vi "Query Trace Data.vi"(8 "error in (no error)":errorcluster, 10 "Trace Number":u8=1, 11 "VNA-PNA in":refnum<class "VNA-PNA.lvclass">) -> (0 "error out":errorcluster, 1 "Data":dbl[](array[numeric]), 2 "Frequency":dbl[](array[numeric]), 3 "VNA-PNA out":refnum<class "VNA-PNA.lvclass">)   [LabVIEW 2020, in "VNA-PNA.lvclass"]
doc: "Query the active trace data.\nIt returns both x and y data"
uses:
  VNA-PNA.lvclass
  C:/Sandbox/RF Bench/Source Code/WiSpry Test Framework/Instruments/Instrument.lvclass
  C:/Sandbox/RF Bench/Source Code/WiSpry Test Framework/Instruments/Vector Network Analyzer/Vector Network Analyzer.lvclass
  Vector Network Analyzer.lvclass/Vector Network Analyzer.ctl
  Instrument.lvclass/Instrument.ctl
  Instrument.lvclass
  Vector Network Analyzer.lvclass
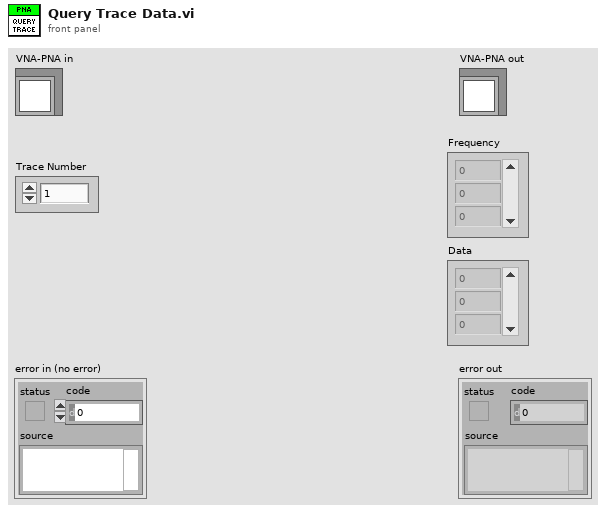
[diagram p1: front panel]
types:
  T1 = enum16{"big-endian, network order", "native, host order", "little-endian"}
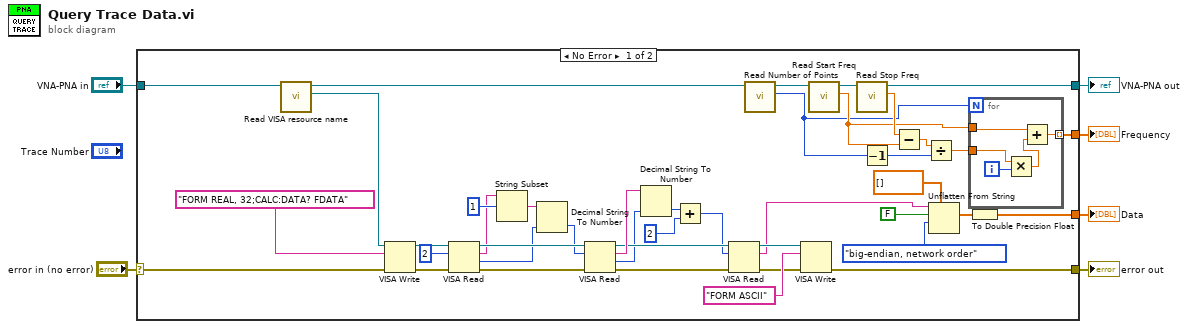
[diagram p0: block diagram]
diagram:
  n1 = case shown="No Error" "error in (no error)" {
    selector: "error in (no error)" -> [w48 w55]
    tunnel: [w29 w55] -> w3
    tunnel: [w36 w54] -> w4
    tunnel: [w31 _] -> w1
    tunnel: [w14 _] -> w2
    tunnel: "VNA-PNA in" -> [w7 w54]
    frame No Error {
      n2 = call "Read VISA resource name.vi"("Instrument in"=w7) -> ("VISA resource name"=w47:refnum<visa-resource-name>, "Instrument out"=w39:refnum<class "VNA-PNA.lvclass">)  [unwired: 9 in]
      n3 = VISA Write(VISA resource name=w47, write buffer="FORM REAL, 32;CALC:DATA? FDATA" ("initial string"), error in (no error)=w48) -> (VISA resource name out=w45:refnum<visa-resource-name>, error out=w46:errorcluster)  [unwired: 1 out]
      n4 = VISA Read(VISA resource name=w45, byte count=u32 2, error in (no error)=w46) -> (VISA resource name out=w42:refnum<visa-resource-name>, read buffer=w20:string, return count=w41:u32, error out=w43:errorcluster)
      n5 = String Subset(string=w20, offset (0)=1) -> (substring=w22:string)  [unwired: 1 in]
      n6 = Decimal String To Number(string=w22, default (0L)=w41) -> (number=w12:u32)  [unwired: 1 in, 1 out]
      n7 = VISA Read(VISA resource name=w42, byte count=w12, error in (no error)=w43) -> (VISA resource name out=w27:refnum<visa-resource-name>, read buffer=w28:string, return count=w19:u32, error out=w26:errorcluster)
      n8 = Decimal String To Number(string=w28, default (0L)=w19) -> (number=w23:u32)  [unwired: 1 in, 1 out]
      n9 = Add(x=w23, y=u32 2) -> (x+y=w11:u32)
      n10 = VISA Read(VISA resource name=w27, byte count=w11, error in (no error)=w26) -> (VISA resource name out=w24:refnum<visa-resource-name>, read buffer=w18:string, error out=w25:errorcluster)  [unwired: 1 out]
      n11 = call "Read Number of Points.vi"("Vector Network Analyzer in"=w39) -> ("Number of Points"=w8:i32, "Vector Network Analyzer out"=w38:refnum<class "VNA-PNA.lvclass">)  [unwired: 9 in]
      n12 = VISA Write(VISA resource name=w24, write buffer="FORM ASCII", error in (no error)=w25) -> (error out=w29:errorcluster)  [unwired: 2 out]
      n13 = call "Read Start Freq.vi"("Vector Network Analyzer in"=w38) -> ("Start Freq"=w33:dbl, "Vector Network Analyzer out"=w37:refnum<class "VNA-PNA.lvclass">)  [unwired: 9 in]
      n14 = call "Read Stop Freq.vi"("Vector Network Analyzer in"=w37) -> ("Stop Freq"=w35:dbl, "Vector Network Analyzer out"=w36:refnum<class "VNA-PNA.lvclass">)  [unwired: 9 in]
      n15 = Decrement(x=w8) -> (x-1=w9:i32)
      n16 = Subtract(x=w35, y=w33) -> (x-y=w34:dbl)
      n17 = Divide(x=w34, y=w9) -> (x/y=w32:dbl)
      n18 = Unflatten From String(type=sgl[] [], binary string=w18, data includes array or string size? (T)=FALSE, byte order (0:big-endian, network order)=T1."big-endian, network order") -> (value=w15:sgl[])  [unwired: 1 in, 2 out]
      n19 = for {
        N: w8 -> [_]
        tunnel: w33 -> [w50]
        tunnel: w32 -> [w52]
        tunnel: [w49] -> w31 mode=indexing
        i -> [w53]
        n20 = Multiply(x=w52, y=w53) -> (x*y=w51:dbl)
        n21 = Add(x=w50, y=w51) -> (x+y=w49:dbl)
      }
      n22 = To Double Precision Float(number=w15) -> (double precision float=w14:dbl[])
    }
    frame Error {
    }
  }
  "error out" <- w3
  "VNA-PNA out" <- w4
  "Data" <- w2
  "Frequency" <- w1
